vi "Initialise ctrl states.vi"(8 "error in (no error)":errorcluster) -> (0 "error out":errorcluster)   [LabVIEW 2013]
uses:
  Typedefs/HW config states enum.ctl
  Global Variables/gl_UI Ctrl Refs.vi
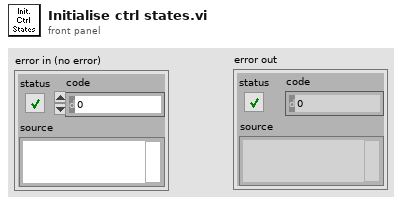
[diagram p1: front panel]
types:
  T1 = enum8{"Enabled", "Disabled", "Disabled and Grayed Out"}
  T2 = typedef "UI ctrl refs cluster.ctl" = cluster{"Top level VI path":path, "Top level VI ref":refnum<vi>, "User menu ref":refnum<k9>, "Sub Panel control":refnum<vi>, "Imaging Param Tab":refnum<vi>, "Occurrence-Start drivers":refnum<k4>, "Occurrence-Speed logging initialised":refnum<k4>, "Occurrence-XYZ stage initialised":refnum<k4>, "Exit button":refnum<vi>, "Status ind":refnum<vi>, "Return to Origin":refnum<vi>, "Speed Logging":refnum<vi>, "Time Lapse":refnum<vi>, "Live Imaging":refnum<vi>, "AOL Z Stack":refnum<vi>, "Motor Z Stack":refnum<vi>, "Funct Acq button":refnum<vi>, "Hard Shutter":refnum<vi>, "Virtual Shutter":refnum<vi>, "Laser Power":refnum<vi>, "AOL Mode":refnum<vi>, "Frame Size":refnum<vi>, "Field of View":refnum<vi>, "Dwell Time":refnum<vi>, "Zoom":refnum<vi>, "AOL Z":refnum<vi>, "Objective":refnum<vi>, "Axis":refnum<vi>, "Paths & Names":refnum<vi>, "Experiment folder path (ind.)":refnum<vi>, "Last State (Ind.)":refnum<vi>, "Laser wavelength ind (nm)":refnum<vi>, "Averages":refnum<vi>, "Angle (degrees)":refnum<vi>, "X centre":refnum<vi>, "Y centre":refnum<vi>, "Plane Mode":refnum<vi>, "# Planes":refnum<vi>, "Z Start":refnum<vi>, "Z Stop":refnum<vi>, "Z Step":refnum<vi>, "PMT 1":refnum<vi>, "PMT 2":refnum<vi>, "Stage XYZ Position":refnum<vi>, "Pockels@Z Start":refnum<vi>, "Pockels@Z Stop":refnum<vi>, "Obtain Z Start":refnum<vi>, "Obtain Z Stop":refnum<vi>, "Live stim.trig.period":refnum<vi>, "Live stim.trig.enable":refnum<vi>, "Funct. Acq. Pockels Modulation":refnum<vi>, "Enable Video Recording":refnum<vi>, "Video Record-Live Imaging":refnum<vi>, "Video Record-Funct acq":refnum<vi>, "AOL Z-stack Chirps Ready (ind)":refnum<vi>, "Center freq ind (nm)":refnum<vi>, "Logging queue (ind)":refnum<vi>, "Back aperture power (ind.)":refnum<vi>, "Power after objective (ind.)":refnum<vi>, "Switch user":refnum<vi>}
  T3 = typedef "HW config states enum.ctl" = enum16{"Load from file", "Save to file", "Write all", "Read all", "Write XY stage settings", "Write DAQ FPGA settings", "Write Control FPGA settings", "Write Phys Channels", "Clear", "Compare from file"}
  T4 = typedef "Sys Configuration.ctl" = cluster{"XY Stage":T5, "DAQ FPGA":T6, "Control system":T10, "Encoder":T11, "DAQmx Chan":T12, "Computer MAC address":string, "Cam VidRec":T13, "Externalise Triggers":bool, "Laser wavelength (nm)":dbl}
  T5 = typedef "XY Stage config cluster.ctl" = cluster{"COM port":refnum<visa-resource-name>, "XY stage available":bool}
  T6 = typedef "DAQ FPGA config cluster.ctl" = cluster{"Ref":T7, "Target":T8, "Clock Freq (MHz) ":dbl, "input card type":T9, "Samples Wait after Trigger":u16, "AOD fill":u16, "StartupDelay":i32, "Slip Cycle (clock cycles)":u32, "Add Cycle":bool}
  T7 = typedef "FPGA Ref.ctl" = refnum<k20>
  T8 = typedef "nirio_resource_hc.ctl" = tag
  T9 = typedef "FPGA input type AC-DC.ctl" = enum16{"AC Card", "DC Card"}
  T10 = typedef "CTRL system config cluster.ctl" = cluster{"Ethernet opened":bool, "Ethernet Port":u32, "Ctrl FPGA available":bool, "Ctrl FPGA Clock (MHz)":dbl, "Ctrl system MAC address":string, "Control system.Network adapter name":string, "AOD 1 Amplitude":i16, "AOD 2 Amplitude":i16, "AOD 3 Amplitude":i16, "AOD 4 Amplitude":i16, "Data Time Interval (ns)":dbl, "T0 (ns)":dbl, "Ta (ns)":dbl}
  T11 = typedef "Encoder config cluster.ctl" = cluster{"IP address":string, "Port":u16, "Encoder available":bool, "Wheel radius (cm)":dbl}
  T12 = typedef "DAQmx physical channels cluster.ctl" = cluster{"Pockels AO":tag, "Hard shutter AO":tag, "PMT AOs":tag, "Power meter AI":tag}
  T13 = typedef "Cam VidRec HW config setup cluster.ctl" = cluster{"DO flag-Video record":tag, "DO flag-Trial start":tag, "VidRec available":bool}
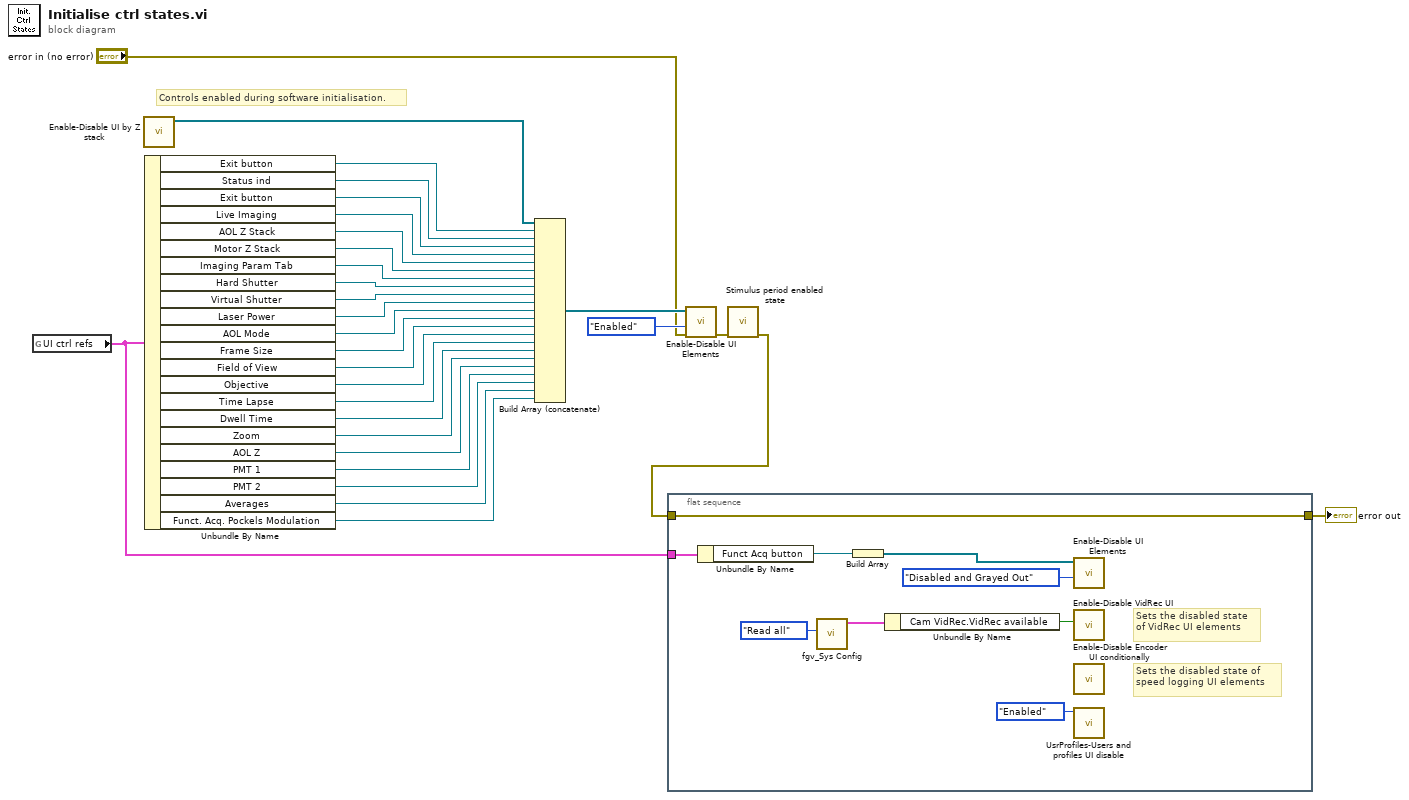
[diagram p0: block diagram]
diagram:
  # "Controls enabled during software initialisation."
  n1 = global read "gl_UI Ctrl Refs.vi" "UI ctrl refs"() -> (w3:T2)
  n2 = call "Enable-Disable UI by Z stack.vi"() -> ("Controls refs to enable/disable"=w4:refnum<vi>[])  [unwired: 11 in]
  n3 = Unbundle By Name(w3) -> ("Exit button"=w8:refnum<vi>, "Status ind"=w12:refnum<vi>, "Exit button"=w13:refnum<vi>, "Live Imaging"=w21:refnum<vi>, "AOL Z Stack"=w20:refnum<vi>, "Motor Z Stack"=w19:refnum<vi>, "Imaging Param Tab"=w30:refnum<vi>, "Hard Shutter"=w28:refnum<vi>, "Virtual Shutter"=w27:refnum<vi>, "Laser Power"=w26:refnum<vi>, "AOL Mode"=w25:refnum<vi>, "Frame Size"=w24:refnum<vi>, "Field of View"=w23:refnum<vi>, "Objective"=w22:refnum<vi>, "Time Lapse"=w17:refnum<vi>, "Dwell Time"=w16:refnum<vi>, "Zoom"=w15:refnum<vi>, "AOL Z"=w14:refnum<vi>, "PMT 1"=w11:refnum<vi>, "PMT 2"=w9:refnum<vi>, "Averages"=w10:refnum<vi>, "Funct. Acq. Pockels Modulation"=w5:refnum<vi>)
  n4 = Build Array (concatenate)(w4, w8, w12, w13, w21, w20, w19, w30, w28, w27, w26, w25, w24, w23, w22, w17, w16, w15, w14, w11, w9, w10, w5) -> (w29:refnum<vi>[])
  n5 = flat-sequence {
    tunnel: w3 -> [w37]
    tunnel: w2 -> [w31]
    tunnel: [w31] -> w1
    frame #0 {
      # "Sets the disabled state of speed logging UI elements"
      # "Sets the disabled state of VidRec UI elements"
      n6 = Unbundle By Name(w37) -> ("Funct Acq button"=w33:refnum<vi>)
      n7 = call "fgv_Sys Config.vi"("Function"=HW_config_states_enum."Read all") -> ("System Config out"=w34:T4)  [unwired: 9 in, 1 out]
      n8 = Build Array(w33) -> (w38:refnum<vi>[])
      n9 = Unbundle By Name(w34) -> ("Cam VidRec.VidRec available"=w35:bool)
      n10 = call "Enable-Disable UI Elements.vi"("Enable/Disable"=T1."Disabled and Grayed Out", "Ctrl ref's"=w38) -> ()  [unwired: 9 in, 1 out]
      n11 = call "Enable-Disable VidRec UI.vi"("Cam VidRec.VidRec available"=w35) -> ()  [unwired: 11 in]
      n12 = call "Enable-Disable Encoder UI conditionally.vi"() -> ()  [unwired: 11 in, 1 out]
      n13 = call "UsrProfiles-Users and profiles UI disable.vi"("Users & Profiles available?"=T1."Enabled") -> ()  [unwired: 10 in, 1 out]
    }
  }
  n14 = call "Enable-Disable UI Elements.vi"("error in (no error)"="error in (no error)", "Enable/Disable"=T1."Enabled", "Ctrl ref's"=w29) -> ("error out"=w7:errorcluster)  [unwired: 8 in]
  n15 = call "Stimulus period enabled state.vi"("error in (no error)"=w7) -> ("error out"=w2:errorcluster)  [unwired: 10 in]
  "error out" <- w1
